vi "rsscope_core_global.vi"() -> ()   [LabVIEW 2014] (continued)
 "Access"=2, "Range Table"="rsscope_rngProtocolI2CRWBit", "Read Callback"="", "Write Callback"="", "Supported Models"="", "Instrument Options"="", "Flags"=0, "Help"="Defines if the R/W bit of a 7-bit address is considered separately or as part of the address.\n\nAvailable Repeated Capabilities:\nSerialBus: SB1, SB2, SB3, SB4\r\n\nRemote-control command(s):\nBUS<m>:I2C:RWBit"}, {"Level"=3, "Class Only"=FALSE, "Identifier"="RSSCOPE_ATTR_PROTOCOL_I2C_SELECTED_FRAME", "Descriptive Name"="Protocol I2C Selected Frame", "Data Type"=0, "Command"="", "Access"=2, "Range Table"="", "Read Callback"="", "Write Callback"="", "Supported Models"="", "Instrument Options"="", "Flags"=0, "Help"="Sets selector repeated capability Frame.\n\nAvailable Repeated Capabilities:\nNone\n\nRemote-control command(s):\ncmd"}, {"Level"=3, "Class Only"=FALSE, "Identifier"="RSSCOPE_ATTR_PROTOCOL_I2C_FRAME_COUNT", "Descriptive Name"="Protocol I2C Frame Count", "Data Type"=0, "Command"="BUS{SerialBus}:I2C:FCO?", "Access"=0, "Range Table"="", "Read Callback"="", "Write Callback"="", "Supported Models"="", "Instrument Options"="K0|K1", "Flags"=0, "Help"="Returns the number of decoded frames.\n\nAvailable Repeated Capabilities:\nSerialBus: SB1, SB2, SB3, SB4\r\n\nRemote-control command(s):\nBUS<m>:I2C:FCOunt?"}, {"Level"=3, "Class Only"=FALSE, "Identifier"="RSSCOPE_ATTR_PROTOCOL_I2C_FRAME_STATUS", "Descriptive Name"="Protocol I2C Frame Status", "Data Type"=0, "Command"="BUS{SerialBus}:I2C:FRAM<Frame>:STAT?", "Access"=0, "Range Table"="RsScope_rngI2CFrameStatus", "Read Callback"="rsscope_FormatI2CFrameRepCapInt32_ReadCallback.vi", "Write Callback"="", "Supported Models"="", "Instrument Options"="K1", "Flags"=0, "Help"="The overall state of the frame.\n\nAvailable Repeated Capabilities:\nSerialBus: SB1, SB2, SB3, SB4\r\n\nRemote-control command(s):\nBUS<m>:I2C:FRAMe<n>:STATus?"}, {"Level"=3, "Class Only"=FALSE, "Identifier"="RSSCOPE_ATTR_PROTOCOL_I2C_FRAME_START", "Descriptive Name"="Protocol I2C Frame Start", "Data Type"=1, "Command"="BUS{SerialBus}:I2C:FRAM<Frame>:STAR?", "Access"=0, "Range Table"="", "Read Callback"="rsscope_FormatI2CFrameRepCapReal64_ReadCallback.vi", "Write Callback"="", "Supported Models"="", "Instrument Options"="K1", "Flags"=0, "Help"="Return the start time of the selected frame.\n\nAvailable Repeated Capabilities:\nSerialBus: SB1, SB2, SB3, SB4\r\n\nRemote-control command(s):\nBUS<m>:I2C:FRAMe<n>:STARt?"}, {"Level"=3, "Class Only"=FALSE, "Identifier"="RSSCOPE_ATTR_PROTOCOL_I2C_FRAME_STOP", "Descriptive Name"="Protocol I2C Frame Stop", "Data Type"=1, "Command"="BUS{SerialBus}:I2C:FRAM<Frame>:STOP?", "Access"=0, "Range Table"="", "Read Callback"="rsscope_FormatI2CFrameRepCapReal64_ReadCallback.vi", "Write Callback"="", "Supported Models"="", "Instrument Options"="K1", "Flags"=0, "Help"="Return the stop time of the selected frame.\n\nAvailable Repeated Capabilities:\nSerialBus: SB1, SB2, SB3, SB4\r\n\nRemote-control command(s):\nBUS<m>:I2C:FRAMe<n>:STOP?"}, {"Level"=3, "Class Only"=FALSE, "Identifier"="RSSCOPE_ATTR_PROTOCOL_I2C_FRAME_ADDRESS_TYPE", "Descriptive Name"="Protocol I2C Frame Address Type", "Data Type"=0, "Command"="BUS{SerialBus}:I2C:FRAM<Frame>:AMOD?", "Access"=0, "Range Table"="RsScope_rngI2CFrameAddressType", "Read Callback"="rsscope_FormatI2CFrameRepCapInt32_ReadCallback.vi", "Write Callback"="", "Supported Models"="", "Instrument Options"="K1", "Flags"=0, "Help"="Returns the address length.\n\nAvailable Repeated Capabilities:\nSerialBus: SB1, SB2, SB3, SB4\r\n\nRemote-control command(s):\nBUS<m>:I2C:FRAMe<n>:AMODe?"}, {"Level"=3, "Class Only"=FALSE, "Identifier"="RSSCOPE_ATTR_PROTOCOL_I2C_FRAME_ADDRESS", "Descriptive Name"="Protocol I2C Frame Address", "Data Type"=0, "Command"="BUS{SerialBus}:I2C:FRAM<Frame>:ADDR?", "Access"=0, "Range Table"="", "Read Callback"="rsscope_FormatI2CFrameRepCapInt32_ReadCallback.vi", "Write Callback"="", "Supported Models"="", "Instrument Options"="K1", "Flags"=0, "Help"="Value of the frame address.\n\nAvailable Repeated Capabilities:\nSerialBus: SB1, SB2, SB3, SB4\r\n\nRemote-control command(s):\nBUS<m>:I2C:FRAMe<n>:ADDRess?"}, {"Level"=3, "Class Only"=FALSE, "Identifier"="RSSCOPE_ATTR_PROTOCOL_I2C_FRAME_RW_BIT", "Descriptive Name"="Protocol I2C Frame RW Bit", "Data Type"=0, "Command"="BUS{SerialBus}:I2C:FRAM<Frame>:ACC?", "Access"=0, "Range Table"="RsScope_rngI2CFrameRWBit", "Read Callback"="rsscope_FormatI2CFrameRepCapInt32_ReadCallback.vi", "Write Callback"="", "Supported Models"="", "Instrument Options"="K1", "Flags"=0, "Help"="Value of the R/W bit.\n\nAvailable Repeated Capabilities:\nSerialBus: SB1, SB2, SB3, SB4\r\n\nRemote-control command(s):\nBUS<m>:I2C:FRAMe<n>:ACCess?"}, {"Level"=3, "Class Only"=FALSE, "Identifier"="RSSCOPE_ATTR_PROTOCOL_I2C_FRAME_ACK_BIT", "Descriptive Name"="Protocol I2C Frame Ack Bit", "Data Type"=0, "Command"="BUS{SerialBus}:I2C:FRAM<Frame>:AACC?", "Access"=0, "Range Table"="RsScope_rngI2CFrameAckBit", "Read Callback"="rsscope_FormatI2CFrameRepCapInt32_ReadCallback.vi", "Write Callback"="", "Supported Models"="", "Instrument Options"="K1", "Flags"=0, "Help"="Value of the address acknowledge bit.\n\nAvailable Repeated Capabilities:\nSerialBus: SB1, SB2, SB3, SB4\r\n\nRemote-control command(s):\nBUS<m>:I2C:FRAMe<n>:AACCess?"}, {"Level"=3, "Class Only"=FALSE, "Identifier"="RSSCOPE_ATTR_PROTOCOL_I2C_FRAME_ACCESS_BIT_START", "Descriptive Name"="Protocol I2C Frame Access Bit Start", "Data Type"=1, "Command"="BUS{SerialBus}:I2C:FRAM<Frame>:RWBS?", "Access"=0, "Range Table"="", "Read Callback"="rsscope_FormatI2CFrameRepCapReal64_ReadCallback.vi", "Write Callback"="", "Supported Models"="", "Instrument Options"="K1", "Flags"=0, "Help"="Queries the start time of the access ack bit.\n\nAvailable Repeated Capabilities:\nSerialBus: SB1, SB2, SB3, SB4\r\n\nRemote-control command(s):\nBUS<m>:I2C:FRAMe<n>:RWBStart?"}, {"Level"=3, "Class Only"=FALSE, "Identifier"="RSSCOPE_ATTR_PROTOCOL_I2C_FRAME_SLAVE_ADDRESS", "Descriptive Name"="Protocol I2C Frame Slave Address", "Data Type"=0, "Command"="BUS{SerialBus}:I2C:FRAM<Frame>:ADEV?", "Access"=0, "Range Table"="", "Read Callback"="rsscope_FormatI2CFrameRepCapInt32_ReadCallback.vi", "Write Callback"="", "Supported Models"="", "Instrument Options"="K1", "Flags"=0, "Help"="Queries the slave address of the indicated frame.\n\nAvailable Repeated Capabilities:\nSerialBus: SB1, SB2, SB3, SB4\r\n\nRemote-control command(s):\nBUS<m>:I2C:FRAMe<n>:ADEVice?"}, {"Level"=3, "Class Only"=FALSE, "Identifier"="RSSCOPE_ATTR_PROTOCOL_I2C_FRAME_ADDRESS_START", "Descriptive Name"="Protocol I2C Frame Address Start", "Data Type"=1, "Command"="BUS{SerialBus}:I2C:FRAM<Frame>:AST?", "Access"=0, "Range Table"="", "Read Callback"="rsscope_FormatI2CFrameRepCapReal64_ReadCallback.vi", "Write Callback"="", "Supported Models"="", "Instrument Options"="K1", "Flags"=0, "Help"="Queries the start time of the address field for the indicated frame.\n\nAvailable Repeated Capabilities:\nSerialBus: SB1, SB2, SB3, SB4\r\n\nRemote-control command(s):\nBUS<m>:I2C:FRAMe<n>:ASTart?"}, {"Level"=3, "Class Only"=FALSE, "Identifier"="RSSCOPE_ATTR_PROTOCOL_I2C_FRAME_ADDRESS_ACK_BIT_START", "Descriptive Name"="Protocol I2C Frame Address Ack Bit Start", "Data Type"=1, "Command"="BUS{SerialBus}:I2C:FRAM<Frame>:ADBS?", "Access"=0, "Range Table"="", "Read Callback"="rsscope_FormatI2CFrameRepCapReal64_ReadCallback.vi", "Write Callback"="", "Supported Models"="", "Instrument Options"="K1", "Flags"=0, "Help"="Queries the start time of the address acknowledge bit.\n\nAvailable Repeated Capabilities:\nSerialBus: SB1, SB2, SB3, SB4\r\n\nRemote-control command(s):\nBUS<m>:I2C:FRAMe<n>:ADBStart?"}, {"Level"=3, "Class Only"=FALSE, "Identifier"="RSSCOPE_ATTR_PROTOCOL_I2C_FRAME_ADDRESS_COMPLETE", "Descriptive Name"="Protocol I2C Frame Address Complete", "Data Type"=3, "Command"="BUS{SerialBus}:I2C:FRAM<Frame>:ACOM?", "Access"=0, "Range Table"="", "Read Callback"="rsscope_FormatI2CFrameRepCapBoolean_ReadCallback.vi", "Write Callback"="", "Supported Models"="", "Instrument Options"="K1", "Flags"=0, "Help"="This function checks if address is complete.\n\nAvailable Repeated Capabilities:\nSerialBus: SB1, SB2, SB3, SB4\r\n\nRemote-control command(s):\nBUS<m>:I2C:FRAMe<n>:ACOMplete?"}, {"Level"=3, "Class Only"=FALSE, "Identifier"="RSSCOPE_ATTR_PROTOCOL_I2C_FRAME_BIT_RATE", "Descriptive Name"="Protocol I2C Frame Bit Rate", "Data Type"=5, "Command"="BUS{SerialBus}:I2C:FRAM<Frame>:BITR?", "Access"=0, "Range Table"="", "Read Callback"="rsscope_FormatI2CFrameRepCapInt64_ReadCallback.vi", "Write Callback"="", "Supported Models"="", "Instrument Options"="K1", "Flags"=0, "Help"="Returns the primary bit rate.\n\nAvailable Repeated Capabilities:\nSerialBus: SB1, SB2, SB3, SB4\r\n\nRemote-control command(s):\nBUS<m>:I2C:FRAMe<n>:BITRate?"}, {"Level"=3, "Class Only"=FALSE, "Identifier"="RSSCOPE_ATTR_PROTOCOL_I2C_FRAME_LENGTH", "Descriptive Name"="Protocol I2C Frame Length", "Data Type"=0, "Command"="BUS{SerialBus}:I2C:FRAM<Frame>:BCO?", "Access"=0, "Range Table"="", "Read Callback"="rsscope_FormatI2CFrameRepCapInt32_ReadCallback.vi", "Write Callback"="", "Supported Models"="", "Instrument Options"="K1", "Flags"=0, "Help"="This function returns the number of bytes in the specified frame.\n\nAvailable Repeated Capabilities:\nSerialBus: SB1, SB2, SB3, SB4\r\n\nRemote-control command(s):\nBUS<m>:I2C:FRAMe<n>:BCOunt?"}, {"Level"=3, "Class Only"=FALSE, "Identifier"="RSSCOPE_ATTR_PROTOCOL_I2C_FRAME_LABEL", "Descriptive Name"="Protocol I2C Frame Label", "Data Type"=2, "Command"="BUS{SerialBus}:I2C:FRAM<Frame>:SYMB?", "Access"=0, "Range Table"="", "Read Callback"="rsscope_FormatI2CFrameRepCapString_ReadCallback.vi", "Write Callback"="", "Supported Models"="", "Instrument Options"="K1", "Flags"=0, "Help"="This attribute returns the symbolic label of the specified frame if the label list is enabled.\n\nAvailable Repeated Capabilities:\nSerialBus: SB1, SB2, SB3, SB4\r\n\nRemote-control command(s):\nBUS<m>:I2C:FRAMe<n>:SYMBol?"}, {"Level"=3, "Class Only"=FALSE, "Identifier"="RSSCOPE_ATTR_PROTOCOL_I2C_SELECTED_BYTE", "Descriptive Name"="Protocol I2C Selected Byte", "Data Type"=0, "Command"="", "Access"=2, "Range Table"="", "Read Callback"="", "Write Callback"="", "Supported Models"="", "Instrument Options"="", "Flags"=0, "Help"="Sets selector repeated capability Byte.\n\nAvailable Repeated Capabilities:\nNone\n\nRemote-control command(s):\ncmd"}, {"Level"=3, "Class Only"=FALSE, "Identifier"="RSSCOPE_ATTR_PROTOCOL_I2C_FRAME_BYTE_DATA", "Descriptive Name"="Protocol I2C Frame Byte Data", "Data Type"=0, "Command"="BUS{SerialBus}:I2C:FRAM<Frame>:BYTE<Byte>:VAL?", "Access"=0, "Range Table"="", "Read Callback"="rsscope_FormatI2CByteRepCapInt32_ReadCallback.vi", "Write Callback"="", "Supported Models"="", "Instrument Options"="K1", "Flags"=0, "Help"="Value of the specified byte.\n\nAvailable Repeated Capabilities:\nSerialBus: SB1, SB2, SB3, SB4\r\n\nRemote-control command(s):\nBUS<m>:I2C:FRAMe<n>:BYTE<o>:VALue?"}, {"Level"=3, "Class Only"=FALSE, "Identifier"="RSSCOPE_ATTR_PROTOCOL_I2C_FRAME_BYTE_ACK_BIT_START", "Descriptive Name"="Protocol I2C Frame Byte Ack Bit Start", "Data Type"=1, "Command"="BUS{SerialBus}:I2C:FRAM<Frame>:BYTE<Byte>:ACKS?", "Access"=0, "Range Table"="", "Read Callback"="rsscope_FormatI2CByteRepCapReal64_ReadCallback.vi", "Write Callback"="", "Supported Models"="", "Instrument Options"="K1", "Flags"=0, "Help"="Returns the start time of the acknowledge bit of the specified byte.\n\nAvailable Repeated Capabilities:\nSerialBus: SB1, SB2, SB3, SB4\r\n\nRemote-control command(s):\nBUS<m>:I2C:FRAMe<n>:BYTE<o>:ACKStart?"}, {"Level"=3, "Class Only"=FALSE, "Identifier"="RSSCOPE_ATTR_PROTOCOL_I2C_FRAME_BYTE_START", "Descriptive Name"="Protocol I2C Frame Byte Start", "Data Type"=1, "Command"="BUS{SerialBus}:I2C:FRAM<Frame>:BYTE<Byte>:STAR?", "Access"=0, "Range Table"="", "Read Callback"="rsscope_FormatI2CByteRepCapReal64_ReadCallback.vi", "Write Callback"="", "Supported Models"="", "Instrument Options"="K1", "Flags"=0, "Help"="Queries the start time of the specified data byte.\n\nAvailable Repeated Capabilities:\nSerialBus: SB1, SB2, SB3, SB4\r\n\nRemote-control command(s):\nBUS<m>:I2C:FRAMe<n>:BYTE<o>:STARt?"}, {"Level"=3, "Class Only"=FALSE, "Identifier"="RSSCOPE_ATTR_PROTOCOL_I2C_FRAME_BYTE_ACK_BIT", "Descriptive Name"="Protocol I2C Frame Byte Ack Bit", "Data Type"=0, "Command"="BUS{SerialBus}:I2C:FRAM<Frame>:BYTE<Byte>:ACC?", "Access"=0, "Range Table"="RsScope_rngI2CFrameAckBit", "Read Callback"="rsscope_FormatI2CByteRepCapInt32_ReadCallback.vi", "Write Callback"="", "Supported Models"="", "Instrument Options"="K1", "Flags"=0, "Help"="Returns the acknowledge bit value of the specified data byte.\n\nAvailable Repeated Capabilities:\nSerialBus: SB1, SB2, SB3, SB4\r\n\nRemote-control command(s):\nBUS<m>:I2C:FRAMe<n>:BYTE<o>:ACCess?"}, {"Level"=3, "Class Only"=FALSE, "Identifier"="RSSCOPE_ATTR_PROTOCOL_I2C_FRAME_BYTE_COMPLETE", "Descriptive Name"="Protocol I2C Frame Byte Complete", "Data Type"=3, "Command"="BUS{SerialBus}:I2C:FRAM<Frame>:BYTE<Byte>:COMP?", "Access"=0, "Range Table"="", "Read Callback"="rsscope_FormatI2CByteRepCapBoolean_ReadCallback.vi", "Write Callback"="", "Supported Models"="", "Instrument Options"="K1", "Flags"=0, "Help"="Returns if the indicated byte is completely contained in the acquisition.\n\nAvailable Repeated Capabilities:\nSerialBus: SB1, SB2, SB3, SB4\r\n\nRemote-control command(s):\nBUS<m>:I2C:FRAMe<n>:BYTE<o>:COMPlete?"}, {"Level"=3, "Class Only"=TRUE, "Identifier"="", "Descriptive Name"="SCL", "Data Type"=0, "Command"="", "Access"=0, "Range Table"="", "Read Callback"="", "Write Callback"="", "Supported Models"="", "Instrument Options"="", "Flags"=0, "Help"="Configures I2C SCL properties."}, {"Level"=4, "Class Only"=FALSE, "Identifier"="RSSCOPE_ATTR_PROTOCOL_I2C_SCL_SOURCE", "Descriptive Name"="Protocol I2C SCL Source", "Data Type"=0, "Command"="BUS{SerialBus}:I2C:SCL:SOUR", "Access"=2, "Range Table"="rsscope_rngProtocolWaveformSource", "Read Callback"="", "Write Callback"="", "Supported Models"="", "Instrument Options"="", "Flags"=0, "Help"="Sets the waveform of the clock line.\n\nAvailable Repeated Capabilities:\nSerialBus: SB1, SB2, SB3, SB4\r\n\nRemote-control command(s):\nBUS<m>:I2C:SCL:SOURce"}, {"Level"=4, "Class Only"=FALSE, "Identifier"="RSSCOPE_ATTR_PROTOCOL_I2C_SCL_THRESHOLD", "Descriptive Name"="Protocol I2C SCL Threshold", "Data Type"=1, "Command"="BUS{SerialBus}:I2C:SCL:THR", "Access"=2, "Range Table"="rsscope_rngProtocolThreshold", "Read Callback"="", "Write Callback"="", "Supported Models"="", "Instrument Options"="", "Flags"=0, "Help"="Sets a user-defined threshold value for the clock line.\n\nAvailable Repeated Capabilities:\nSerialBus: SB1, SB2, SB3, SB4\r\n\nRemote-control command(s):\nBUS<m>:I2C:SCL:THReshold"}, {"Level"=3, "Class Only"=TRUE, "Identifier"="", "Descriptive Name"="SDA", "Data Type"=0, "Command"="", "Access"=0, "Range Table"="", "Read Callback"="", "Write Callback"="", "Supported Models"="", "Instrument Options"="", "Flags"=0, "Help"="Configures I2C SDA properties."}, {"Level"=4, "Class Only"=FALSE, "Identifier"="RSSCOPE_ATTR_PROTOCOL_I2C_SDA_SOURCE", "Descriptive Name"="Protocol I2C SDA Source", "Data Type"=0, "Command"="BUS{SerialBus}:I2C:SDA:SOUR", "Access"=2, "Range Table"="rsscope_rngProtocolWaveformSource", "Read Callback"="", "Write Callback"="", "Supported Models"="", "Instrument Options"="", "Flags"=0, "Help"="Sets the waveform of the data line.\n\nAvailable Repeated Capabilities:\nSerialBus: SB1, SB2, SB3, SB4\r\n\nRemote-control command(s):\nBUS<m>:I2C:SDA:SOURce"}, {"Level"=4, "Class Only"=FALSE, "Identifier"="RSSCOPE_ATTR_PROTOCOL_I2C_SDA_THRESHOLD", "Descriptive Name"="Protocol I2C SDA Threshold", "Data Type"=1, "Command"="BUS{SerialBus}:I2C:SDA:THR", "Access"=2, "Range Table"="rsscope_rngProtocolThreshold", "Read Callback"="", "Write Callback"="", "Supported Models"="", "Instrument Options"="", "Flags"=0, "Help"="Sets a user-defined threshold value for the data line.\n\nAvailable Repeated Capabilities:\nSerialBus: SB1, SB2, SB3, SB4\r\n\nRemote-control command(s):\nBUS<m>:I2C:SDA:THReshold"}, {"Level"=2, "Class Only"=TRUE, "Identifier"="", "Descriptive Name"="SPI", "Data Type"=0, "Command"="", "Access"=0, "Range Table"="", "Read Callback"="", "Write Callback"="", "Supported Models"="", "Instrument Options"="", "Flags"=0, "Help"="SPI (Serial Peripheral Interface) - decoding requires option R&S RTO-K1"}, {"Level"=3, "Class Only"=FALSE, "Identifier"="RSSCOPE_ATTR_PROTOCOL_SPI_BIT_ORDER", "Descriptive Name"="Protocol SPI Bit Order", "Data Type"=0, "Command"="BUS{SerialBus}:SPI:BORD", "Access"=2, "Range Table"="rsscope_rngProtocolSPIBitOrder", "Read Callback"="", "Write Callback"="", "Supported Models"="", "Instrument Options"="", "Flags"=0, "Help"="Defines if the data of the messages starts with msb (most significant bit) or lsb (least\n  significant bit).\n\nAvailable Repeated Capabilities:\nSerialBus: SB1, SB2, SB3, SB4\r\n\nRemote-control command(s):\nBUS<m>:SPI:BORDer"}, {"Level"=3, "Class Only"=FALSE, "Identifier"="RSSCOPE_ATTR_PROTOCOL_SPI_WORD_LENGTH", "Descriptive Name"="Protocol SPI Word Length", "Data Type"=0, "Command"="BUS{SerialBus}:SPI:WSIZ", "Access"=2, "Range Table"="rsscope_rngProtocolSPIWordLength", "Read Callback"="", "Write Callback"="", "Supported Models"="", "Instrument Options"="", "Flags"=0, "Help"="Sets the number of bits in a message.\n\nAvailable Repeated Capabilities:\nSerialBus: SB1, SB2, SB3, SB4\r\n\nRemote-control command(s):\nBUS<m>:SPI:WSIZe"}, {"Level"=3, "Class Only"=FALSE, "Identifier"="RSSCOPE_ATTR_PROTOCOL_SPI_TECHNOLOGY", "Descriptive Name"="Protocol SPI Technology", "Data Type"=0, "Command"="BUS{SerialBus}:SPI:TECH", "Access"=2, "Range Table"="rsscope_rngProtocolTechnology", "Read Callback"="", "Write Callback"="", "Supported Models"="", "Instrument Options"="", "Flags"=0, "Help"="Sets the threshold voltage clock and data lines as defined for various signal technologies.\n\nFor user defined values set to manual and use RSSCOPE_ATTR_PROTOCOL_SPI_THRESHOLD.\n\nAvailable Repeated Capabilities:\nSerialBus: SB1, SB2, SB3, SB4\r\n\nRemote-control command(s):\nBUS<m>:SPI:TECHnology"}, {"Level"=3, "Class Only"=FALSE, "Identifier"="RSSCOPE_ATTR_PROTOCOL_SPI_FRAME_START_CONDITION", "Descriptive Name"="Protocol SPI Frame Start Condition", "Data Type"=0, "Command"="BUS{SerialBus}:SPI:FRC", "Access"=2, "Range Table"="rsscope_rngProtocolSPIFrameStartCond", "Read Callback"="", "Write Callback"="", "Supported Models"="", "Instrument Options"="", "Flags"=0, "Help"="Select if frame start on Slave Select signal or on Clock line timeout defined by RSSCOPE_ATTR_PROTOCOL_SPI_FRAME_START_TIMEOUT\n\nAvailable Repeated Capabilities:\nSerialBus: SB1, SB2, SB3, SB4\r\n\nRemote-control command(s):\nBUS<m>:SPI:FRCondition"}, {"Level"=3, "Class Only"=FALSE, "Identifier"="RSSCOPE_ATTR_PROTOCOL_SPI_FRAME_START_TIMEOUT", "Descriptive Name"="Protocol SPI Frame Start Timeout", "Data Type"=1, "Command"="BUS{SerialBus}:SPI:TIM", "Access"=2, "Range Table"="rsscope_rngProtocolSPIFrameStartTimeout", "Read Callback"="", "Write Callback"="", "Supported Models"="", "Instrument Options"="", "Flags"=0, "Help"="Sets a timeout on the clock line SCLK as limiter between two frames.\n\nAvailable Repeated Capabilities:\nSerialBus: SB1, SB2, SB3, SB4\r\n\nRemote-control command(s):\nBUS<m>:SPI:TIMeout"}, {"Level"=3, "Class Only"=FALSE, "Identifier"="RSSCOPE_ATTR_PROTOCOL_SPI_SELECTED_FRAME", "Descriptive Name"="Protocol SPI Selected Frame", "Data Type"=0, "Command"="", "Access"=2, "Range Table"="", "Read Callback"="", "Write Callback"="", "Supported Models"="", "Instrument Options"="", "Flags"=0, "Help"="Sets selector repeated capability Frame.\n\nAvailable Repeated Capabilities:\nNone\n\nRemote-control command(s):\ncmd"}, {"Level"=3, "Class Only"=FALSE, "Identifier"="RSSCOPE_ATTR_PROTOCOL_SPI_FRAME_COUNT", "Descriptive Name"="Protocol SPI Frame Count", "Data Type"=0, "Command"="BUS{SerialBus}:SPI:FCOunt?", "Access"=0, "Range Table"="", "Read Callback"="", "Write Callback"="", "Supported Models"="", "Instrument Options"="K0|K1", "Flags"=0, "Help"="Returns the number of decoded frames.\n\nAvailable Repeated Capabilities:\nSerialBus: SB1, SB2, SB3, SB4\r\n\nRemote-control command(s):\nBUS<m>:SPI:FCOunt?"}, {"Level"=3, "Class Only"=FALSE, "Identifier"="RSSCOPE_ATTR_PROTOCOL_SPI_FRAME_WORD_COUNT", "Descriptive Name"="Protocol SPI Frame Word Count", "Data Type"=0, "Command"="BUS{SerialBus}:SPI:FRAM<Frame>:WCO?", "Access"=0, "Range Table"="", "Read Callback"="rsscope_FormatSPIFrameRepCapInt32_ReadCallback.vi", "Write Callback"="", "Supported Models"="", "Instrument Options"="K1", "Flags"=0, "Help"="Queries the number of words in frame.\n\nAvailable Repeated Capabilities:\nSerialBus: SB1, SB2, SB3, SB4\r\n\nRemote-control command(s):\nBUS<m>:SPI:FRAMe<n>:WCOunt?"}, {"Level"=3, "Class Only"=FALSE, "Identifier"="RSSCOPE_ATTR_PROTOCOL_SPI_FRAME_START", "Descriptive Name"="Protocol SPI Frame Start", "Data Type"=1, "Command"="BUS{SerialBus}:SPI:FRAM<Frame>:STAR?", "Access"=0, "Range Table"="", "Read Callback"="rsscope_FormatSPIFrameRepCapReal64_ReadCallback.vi", "Write Callback"="", "Supported Models"="", "Instrument Options"="K1", "Flags"=0, "Help"="Return the start time of the selected frame.\n\nAvailable Repeated Capabilities:\nSerialBus: SB1, SB2, SB3, SB4\r\n\nRemote-control command(s):\nBUS<m>:SPI:FRAMe<n>:STARt?"}, {"Level"=3, "Class Only"=FALSE, "Identifier"="RSSCOPE_ATTR_PROTOCOL_SPI_FRAME_STOP", "Descriptive Name"="Protocol SPI Frame Stop", "Data Type"=1, "Command"="BUS{SerialBus}:SPI:FRAM<Frame>:STOP?", "Access"=0, "Range Table"="", "Read Callback"="rsscope_FormatSPIFrameRepCapReal64_ReadCallback.vi", "Write Callback"="", "Supported Models"="", "Instrument Options"="K1", "Flags"=0, "Help"="Return the stop time of the selected frame.\n\nAvailable Repeated Capabilities:\nSerialBus: SB1, SB2, SB3, SB4\r\n\nRemote-control command(s):\nBUS<m>:SPI:FRAMe<n>:STOP?"}, {"Level"=3, "Class Only"=FALSE, "Identifier"="RSSCOPE_ATTR_PROTOCOL_SPI_FRAME_BIT_RATE", "Descriptive Name"="Protocol SPI Frame Bit Rate", "Data Type"=5, "Command"="BUS{SerialBus}:SPI:FRAM<Frame>:BITR?", "Access"=0, "Range Table"="", "Read Callback"="rsscope_FormatSPIFrameRepCapInt64_ReadCallback.vi", "Write Callback"="", "Supported Models"="", "Instrument Options"="", "Flags"=0, "Help"="Returns the primary bit rate.\n\nAvailable Repeated Capabilities:\nSerialBus: SB1, SB2, SB3, SB4\r\n\nRemote-control command(s):\nBUS<m>:SPI:FRAMe<n>:BITRate?"}, {"Level"=3, "Class Only"=FALSE, "Identifier"="RSSCOPE_ATTR_PROTOCOL_SPI_FRAME_STATUS", "Descriptive Name"="Protocol SPI Frame Status", "Data Type"=0, "Command"="BUS{SerialBus}:SPI:FRAM<Frame>:STAT?", "Access"=0, "Range Table"="RsScope_rngSPIFrameStatus", "Read Callback"="rsscope_FormatSPIFrameRepCapInt32_ReadCallback.vi", "Write Callback"="", "Supported Models"="", "Instrument Options"="K1", "Flags"=0, "Help"="The overall state of the frame.\n\nAvailable Repeated Capabilities:\nSerialBus: SB1, SB2, SB3, SB4\r\n\nRemote-control command(s):\nBUS<m>:SPI:FRAMe<n>:STATus?"}, {"Level"=3, "Class Only"=FALSE, "Identifier"="RSSCOPE_ATTR_PROTOCOL_SPI_SELECTED_WORD", "Descriptive Name"="Protocol SPI Selected Word", "Data Type"=0, "Command"="", "Access"=2, "Range Table"="", "Read Callback"="", "Write Callback"="", "Supported Models"="", "Instrument Options"="", "Flags"=0, "Help"="Sets selector repeated capability Word.\n\nAvailable Repeated Capabilities:\nNone\n\nRemote-control command(s):\ncmd"}, {"Level"=3, "Class Only"=FALSE, "Identifier"="RSSCOPE_ATTR_PROTOCOL_SPI_FRAME_WORD_START", "Descriptive Name"="Protocol SPI Frame Word Start", "Data Type"=1, "Command"="BUS{SerialBus}:SPI:FRAM<Frame>:WORD<Word>:STAR?", "Access"=0, "Range Table"="", "Read Callback"="rsscope_FormatSPIWordRepCapReal64_ReadCallback.vi", "Write Callback"="", "Supported Models"="", "Instrument Options"="K1", "Flags"=0, "Help"="Start time of the data word.\n\nAvailable Repeated Capabilities:\nSerialBus: SB1, SB2, SB3, SB4\r\n\nRemote-control command(s):\nBUS<m>:SPI:FRAMe<n>:WORD<o>:STARt?"}, {"Level"=3, "Class Only"=FALSE, "Identifier"="RSSCOPE_ATTR_PROTOCOL_SPI_FRAME_WORD_STOP", "Descriptive Name"="Protocol SPI Frame Word Stop", "Data Type"=1, "Command"="BUS{SerialBus}:SPI:FRAM<Frame>:WORD<Word>:STOP?", "Access"=0, "Range Table"="", "Read Callback"="rsscope_FormatSPIWordRepCapReal64_ReadCallback.vi", "Write Callback"="", "Supported Models"="", "Instrument Options"="K1", "Flags"=0, "Help"="Stop time of the data word.\n\nAvailable Repeated Capabilities:\nSerialBus: SB1, SB2, SB3, SB4\r\n\nRemote-control command(s):\nBUS<m>:SPI:FRAMe<n>:WORD<o>:STOP?"}, {"Level"=3, "Class Only"=FALSE, "Identifier"="RSSCOPE_ATTR_PROTOCOL_SPI_FRAME_WORD_MISO", "Descriptive Name"="Protocol SPI Frame Word MISO", "Data Type"=0, "Command"="BUS{SerialBus}:SPI:FRAM<Frame>:WORD<Word>:MISO?", "Access"=0, "Range Table"="", "Read Callback"="rsscope_FormatSPIWordRepCapInt32_ReadCallback.vi", "Write Callback"="", "Supported Models"="", "Instrument Options"="K1", "Flags"=0, "Help"="Returns the data value of the specified word on the MISO line.\n\nAvailable Repeated Capabilities:\nSerialBus: SB1, SB2, SB3, SB4\r\n\nRemote-control command(s):\nBUS<m>:SPI:FRAMe<n>:WORD<o>:MISO?"}, {"Level"=3, "Class Only"=FALSE, "Identifier"="RSSCOPE_ATTR_PROTOCOL_SPI_FRAME_WORD_MISO_FORMATTED_VALUE", "Descriptive Name"="Protocol SPI Frame Word MISO Formatted Value", "Data Type"=2, "Command"="BUS{SerialBus}:SPI:FRAM<Frame>:WORD<Word>:FMIS?", "Access"=0, "Range Table"="", "Read Callback"="rsscope_FormatSPIWordRepCapString_ReadCallback.vi", "Write Callback"="", "Supported Models"="", "Instrument Options"="K1", "Flags"=0, "Help"="Returns the formatted value of the specified word on the MISO line.\n\nAvailable Repeated Capabilities:\nSerialBus: SB1, SB2, SB3, SB4\r\n\nRemote-control command(s):\nBUS<m>:SPI:FRAMe<n>:WORD<o>:FMISo?"}, {"Level"=3, "Class Only"=FALSE, "Identifier"="RSSCOPE_ATTR_PROTOCOL_SPI_FRAME_WORD_MOSI", "Descriptive Name"="Protocol SPI Frame Word MOSI", "Data Type"=0, "Command"="BUS{SerialBus}:SPI:FRAM<Frame>:WORD<Word>:MOSI?", "Access"=0, "Range Table"="", "Read Callback"="rsscope_FormatSPIWordRepCapInt32_ReadCallback.vi", "Write Callback"="", "Supported Models"="", "Instrument Options"="K1", "Flags"=0, "Help"="Returns the data value of the specified word on the MOSI line.\n\nAvailable Repeated Capabilities:\nSerialBus: SB1, SB2, SB3, SB4\r\n\nRemote-control command(s):\nBUS<m>:SPI:FRAMe<n>:WORD<o>:MOSI?"}, {"Level"=3, "Class Only"=FALSE, "Identifier"="RSSCOPE_ATTR_PROTOCOL_SPI_FRAME_WORD_MOSI_FORMATTED_VALUE", "Descriptive Name"="Protocol SPI Frame Word MOSI Formatted Value", "Data Type"=2, "Command"="BUS{SerialBus}:SPI:FRAM<Frame>:WORD<Word>:FMOS?", "Access"=0, "Range Table"="", "Read Callback"="rsscope_FormatSPIWordRepCapString_ReadCallback.vi", "Write Callback"="", "Supported Models"="", "Instrument Options"="K1", "Flags"=0, "Help"="Returns the formatted value of the specified word on the MOSI line.\n\nAvailable Repeated Capabilities:\nSerialBus: SB1, SB2, SB3, SB4\r\n\nRemote-control command(s):\nBUS<m>:SPI:FRAMe<n>:WORD<o>:FMOSi?"}, {"Level"=3, "Class Only"=TRUE, "Identifier"="", "Descriptive Name"="Clock", "Data Type"=0, "Command"="", "Access"=0, "Range Table"="", "Read Callback"="", "Write Callback"="", "Supported Models"="", "Instrument Options"="", "Flags"=0, "Help"="Configures SPI Clock properties."}, {"Level"=4, "Class Only"=FALSE, "Identifier"="RSSCOPE_ATTR_PROTOCOL_SPI_CLOCK_SOURCE", "Descriptive Name"="Protocol SPI Clock Source", "Data Type"=0, "Command"="BUS{SerialBus}:SPI:SCLK:SOUR", "Access"=2, "Range Table"="rsscope_rngProtocolWaveformSource", "Read Callback"="", "Write Callback"="", "Supported Models"="", "Instrument Options"="", "Flags"=0, "Help"="Sets the input channel of the clock line.\n\nAvailable Repeated Capabilities:\nSerialBus: SB1, SB2, SB3, SB4\r\n\nRemote-control command(s):\nBUS<m>:SPI:SCLK:SOURce"}, {"Level"=4, "Class Only"=FALSE, "Identifier"="RSSCOPE_ATTR_PROTOCOL_SPI_CLOCK_THRESHOLD", "Descriptive Name"="Protocol SPI Clock Threshold", "Data Type"=1, "Command"="BUS{SerialBus}:SPI:SCLK:THR", "Access"=2, "Range Table"="rsscope_rngProtocolThreshold", "Read Callback"="", "Write Callback"="", "Supported Models"="", "Instrument Options"="", "Flags"=0, "Help"="Set user-defined threshold values for the clock lines.\n\nAvailable Repeated Capabilities:\nSerialBus: SB1, SB2, SB3, SB4\r\n\nRemote-control command(s):\nBUS<m>:SPI:SCLK:THReshold"}, {"Level"=3, "Class Only"=TRUE, "Identifier"="", "Descriptive Name"="MOSI", "Data Type"=0, "Command"="", "Access"=0, "Range Table"="", "Read Callback"="", "Write Callback"="", "Supported Models"="", "Instrument Options"="", "Flags"=0, "Help"="Configures SPI MOSI properties."}, {"Level"=4, "Class Only"=FALSE, "Identifier"="RSSCOPE_ATTR_PROTOCOL_SPI_MOSI_SOURCE", "Descriptive Name"="Protocol SPI MOSI Source", "Data Type"=0, "Command"="BUS{SerialBus}:SPI:MOSI:SOUR", "Access"=2, "Range Table"="rsscope_rngProtocolWaveformSource", "Read Callback"="", "Write Callback"="", "Supported Models"="", "Instrument Options"="", "Flags"=0, "Help"="Sets the input channel of the MOSI line.\n\nAvailable Repeated Capabilities:\nSerialBus: SB1, SB2, SB3, SB4\r\n\nRemote-control command(s):\nBUS<m>:SPI:MOSI:SOURce"}, {"Level"=4, "Class Only"=FALSE, "Identifier"="RSSCOPE_ATTR_PROTOCOL_SPI_MOSI_POLARITY", "Descriptive Name"="Protocol SPI MOSI Polarity", "Data Type"=0, "Command"="BUS{SerialBus}:SPI:MOSI:POL", "Access"=2, "Range Table"="rsscope_rngProtocolSPIPolarity", "Read Callback"="", "Write Callback"="", "Supported Models"="", "Instrument Options"="", "Flags"=0, "Help"="Selects whether transmitted data is high active (high = 1) or low active (low = 1).\n\nAvailable Repeated Capabilities:\nSerialBus: SB1, SB2, SB3, SB4\r\n\nRemote-control command(s):\nBUS<m>:SPI:MOSI:POLarity"}, {"Level"=4, "Class Only"=FALSE, "Identifier"="RSSCOPE_ATTR_PROTOCOL_SPI_MOSI_THRESHOLD", "Descriptive Name"="Protocol SPI MOSI Threshold", "Data Type"=1, "Command"="BUS{SerialBus}:SPI:MOSI:THR", "Access"=2, "Range Table"="rsscope_rngProtocolThreshold", "Read Callback"="", "Write Callback"="", "Supported Models"="", "Instrument Options"="", "Flags"=0, "Help"="Set user-defined threshold values for the MOSI lines.\n\nAvailable Repeated Capabilities:\nSerialBus: SB1, SB2, SB3, SB4\r\n\nRemote-control command(s):\nBUS<m>:SPI:MOSI:THReshold"}, {"Level"=3, "Class Only"=TRUE, "Identifier"="", "Descriptive Name"="MISO", "Data Type"=0, "Command"="", "Access"=0, "Range Table"="", "Read Callback"="", "Write Callback"="", "Supported Models"="", "Instrument Options"="", "Flags"=0, "Help"="Configures SPI MISO properties."}, {"Level"=4, "Class Only"=FALSE, "Identifier"="RSSCOPE_ATTR_PROTOCOL_SPI_MISO_SOURCE", "Descriptive Name"="Protocol SPI MISO Source", "Data Type"=0, "Command"="BUS{SerialBus}:SPI:MISO:SOUR", "Access"=2, "Range Table"="rsscope_rngProtocolWaveformSource", "Read Callback"="", "Write Callback"="", "Supported Models"="", "Instrument Options"="", "Flags"=0, "Help"="Sets the input channel of the MISO line.\n\nAvailable Repeated Capabilities:\nSerialBus: SB1, SB2, SB3, SB4\r\n\nRemote-control command(s):\nBUS<m>:SPI:MISO:SOURce"}, {"Level"=4, "Class Only"=FALSE, "Identifier"="RSSCOPE_ATTR_PROTOCOL_SPI_MISO_POLARITY", "Descriptive Name"="Protocol SPI MISO Polarity", "Data Type"=0, "Command"="BUS{SerialBus}:SPI:MISO:POL", "Access"=2, "Range Table"="rsscope_rngProtocolSPIPolarity", "Read Callback"="", "Write Callback"="", "Supported Models"="", "Instrument Options"="", "Flags"=0, "Help"="Selects whether transmitted data is high active (high = 1) or low active (low = 1).\n\nAvailable Repeated Capabilities:\nSerialBus: SB1, SB2, SB3, SB4\r\n\nRemote-control command(s):\nBUS<m>:SPI:MISO:POLarity"}, {"Level"=4, "Class Only"=FALSE, "Identifier"="RSSCOPE_ATTR_PROTOCOL_SPI_MISO_THRESHOLD", "Descriptive Name"="Protocol SPI MISO Threshold", "Data Type"=1, "Command"="BUS{SerialBus}:SPI:MISO:THR", "Access"=2, "Range Table"="rsscope_rngProtocolThreshold", "Read Callback"="", "Write Callback"="", "Supported Models"="", "Instrument Options"="", "Flags"=0, "Help"="Set user-defined threshold values for the MISO lines.\n\nAvailable Repeated Capabilities:\nSerialBus: SB1, SB2, SB3, SB4\r\n\nRemote-control command(s):\nBUS<m>:SPI:MISO:THReshold"}, {"Level"=3, "Class Only"=TRUE, "Identifier"="", "Descriptive Name"="Slave Select", "Data Type"=0, "Command"="", "Access"=0, "Range Table"="", "Read Callback"="", "Write Callback"="", "Supported Models"="", "Instrument Options"="", "Flags"=0, "Help"="Configures SPI Slave Select properties."}, {"Level"=4, "Class Only"=FALSE, "Identifier"="RSSCOPE_ATTR_PROTOCOL_SPI_SLAVE_SELECT_SOURCE", "Descriptive Name"="Protocol SPI Slave Select Source", "Data Type"=0, "Command"="BUS{SerialBus}:SPI:SSEL:SOUR", "Access"=2, "Range Table"="rsscope_rngProtocolWaveformSource", "Read Callback"="", "Write Callback"="", "Supported Models"="", "Instrument Options"="", "Flags"=0, "Help"="Sets the input channel of the Slave Select line.\n\nAvailable Repeated Capabilities:\nSerialBus: SB1, SB2, SB3, SB4\r\n\nRemote-control command(s):\nBUS<m>:SPI:SSELect:SOURce"}, {"Level"=4, "Class Only"=FALSE, "Identifier"="RSSCOPE_ATTR_PROTOCOL_SPI_SLAVE_SELECT_POLARITY", "Descriptive Name"="Protocol SPI Slave Select Polarity", "Data Type"=0, "Command"="BUS{SerialBus}:SPI:SSEL:POL", "Access"=2, "Range Table"="rsscope_rngProtocolSPIPolarity", "Read Callback"="", "Write Callback"="", "Supported Models"="", "Instrument Options"="", "Flags"=0, "Help"="Selects whether transmitted slave select signal is high active (high = 1) or low active (low = 1).\n\nAvailable Repeated Capabilities:\nSerialBus: SB1, SB2, SB3, SB4\r\n\nRemote-control command(s):\nBUS<m>:SPI:SSELect:POLarity"}, {"Level"=4, "Class Only"=FALSE, "Identifier"="RSSCOPE_ATTR_PROTOCOL_SPI_SLAVE_SELECT_THRESHOLD", "Descriptive Name"="Protocol SPI Slave Select Threshold", "Data Type"=1, "Command"="BUS{SerialBus}:SPI:SSEL:THR", "Access"=2, "Range Table"="rsscope_rngProtocolThreshold", "Read Callback"="", "Write Callback"="", "Supported Models"="", "Instrument Options"="", "Flags"=0, "Help"="Set user-defined threshold values for the slave select lines.\n\nAvailable Repeated Capabilities:\nSerialBus: SB1, SB2, SB3, SB4\r\n\nRemote-control command(s):\nBUS<m>:SPI:SSELect:THReshold"}, {"Level"=2, "Class Only"=TRUE, "Identifier"="", "Descriptive Name"="UART", "Data Type"=0, "Command"="", "Access"=0, "Range Table"="", "Read Callback"="", "Write Callback"="", "Supported Models"="", "Instrument Options"="", "Flags"=0, "Help"="UART/RS232 (EIA-232 serial interface) - decoding requires option R&S RTO-K2"}, {"Level"=3, "Class Only"=FALSE, "Identifier"="RSSCOPE_ATTR_PROTOCOL_UART_TECHNOLOGY", "Descriptive Name"="Protocol UART Technology", "Data Type"=0, "Command"="BUS{SerialBus}:UART:TECH", "Access"=2, "Range Table"="rsscope_rngProtocolTechnology", "Read Callback"="", "Write Callback"="", "Supported Models"="", "Instrument Options"="", "Flags"=0, "Help"="Sets the threshold voltage Tx and Rx lines as defined for various signal technologies.\n\nFor user defined values set to manual and use RSSCOPE_ATTR_PROTOCOL_UART_THRESHOLD.\n\nAvailable Repeated Capabilities:\nSerialBus: SB1, SB2, SB3, SB4\r\n\nRemote-control command(s):\nBUS<m>:UART:TECHnology"}, {"Level"=3, "Class Only"=FALSE, "Identifier"="RSSCOPE_ATTR_PROTOCOL_UART_BIT_RATE", "Descriptive Name"="Protocol UART Bit Rate", "Data Type"=0, "Command"="BUS{SerialBus}:UART:BAUD", "Access"=2, "Range Table"="rsscope_rngProtocolUARTBitRate", "Read Callback"="", "Write Callback"="", "Supported Models"="", "Instrument Options"="", "Flags"=0, "Help"="Sets the number of transmitted bits per second.\n\nAvailable Repeated Capabilities:\nSerialBus: SB1, SB2, SB3, SB4\r\n\nRemote-control command(s):\nBUS<m>:UART:BAUDrate"}, {"Level"=3, "Class Only"=FALSE, "Identifier"="RSSCOPE_ATTR_PROTOCOL_UART_PARITY", "Descriptive Name"="Protocol UART Parity", "Data Type"=0, "Command"="BUS{SerialBus}:UART:PAR", "Access"=2, "Range Table"="rsscope_rngProtocolUARTParity", "Read Callback"="", "Write Callback"="", "Supported Models"="", "Instrument Options"="", "Flags"=0, "Help"="Defines the optional parity bit that is used for error detection.\n\nAvailable Repeated Capabilities:\nSerialBus: SB1, SB2, SB3, SB4\r\n\nRemote-control command(s):\nBUS<m>:UART:PARity"}, {"Level"=3, "Class Only"=FALSE, "Identifier"="RSSCOPE_ATTR_PROTOCOL_UART_POLARITY", "Descriptive Name"="Protocol UART Polarity", "Data Type"=0, "Command"="BUS{SerialBus}:UART:POL", "Access"=2, "Range Table"="rsscope_rngProtocolPolarity", "Read Callback"="", "Write Callback"="", "Supported Models"="", "Instrument Options"="", "Flags"=0, "Help"="Defines if the transmitted data on the bus is high (high = 1) or low (low = 1) active.\n\nAvailable Repeated Capabilities:\nSerialBus: SB1, SB2, SB3, SB4\r\n\nRemote-control command(s):\nBUS<m>:UART:POLarity"}, {"Level"=3, "Class Only"=FALSE, "Identifier"="RSSCOPE_ATTR_PROTOCOL_UART_STOP_BITS", "Descriptive Name"="Protocol UART Stop Bits", "Data Type"=0, "Command"="BUS{SerialBus}:UART:SBIT", "Access"=2, "Range Table"="rsscope_rngProtocolUARTStopBits", "Read Callback"="", "Write Callback"="", "Supported Models"="", "Instrument Options"="", "Flags"=0, "Help"="Sets the number of stop bits: 1; 1.5 or 2 stop bits are possible.\n\nAvailable Repeated Capabilities:\nSerialBus: SB1, SB2, SB3, SB4\r\n\nRemote-control command(s):\nBUS<m>:UART:SBIT"}, {"Level"=3, "Class Only"=FALSE, "Identifier"="RSSCOPE_ATTR_PROTOCOL_UART_DATA_BITS_COUNT", "Descriptive Name"="Protocol UART Data Bits Count", "Data Type"=0, "Command"="BUS{SerialBus}:UART:SSIZ", "Access"=2, "Range Table"="rsscope_rngProtocolUARTDataBitsCount", "Read Callback"="", "Write Callback"="", "Supported Models"="", "Instrument Options"="", "Flags"=0, "Help"="Sets the number of data bits in a message.\n\nAvailable Repeated Capabilities:\nSerialBus: SB1, SB2, SB3, SB4\r\n\nRemote-control command(s):\nBUS<m>:UART:SSIZe"}, {"Level"=3, "Class Only"=FALSE, "Identifier"="RSSCOPE_ATTR_PROTOCOL_UART_WORD_COUNT", "Descriptive Name"="Protocol UART Word Count", "Data Type"=0, "Command"="BUS{SerialBus}:UART:WORD:COUN?", "Access"=0, "Range Table"="", "Read Callback"="", "Write Callback"="", "Supported Models"="", "Instrument Options"="K0|K2", "Flags"=0, "Help"="Returns the number of words in the acquisition.\n\nAvailable Repeated Capabilities:\nSerialBus: SB1, SB2, SB3, SB4\r\n\nRemote-control command(s):\nBUS<m>:UART:WORD<n>:COUNt?"}, {"Level"=3, "Class Only"=FALSE, "Identifier"="RSSCOPE_ATTR_PROTOCOL_UART_PRIMARY_BIT_RATE", "Descriptive Name"="Protocol UART Primary Bit Rate", "Data Type"=5, "Command"="BUS{SerialBus}:UART:WORD1:BITR?", "Access"=0, "Range Table"="", "Read Callback"="", "Write Callback"="", "Supported Models"="", "Instrument Options"="", "Flags"=0, "Help"="Returns the primary bit rate.\n\nAvailable Repeated Capabilities:\nSerialBus: SB1, SB2, SB3, SB4\r\n\nRemote-control command(s):\nBUS<m>:UART:WORD<n>:BITRate?"}, {"Level"=3, "Class Only"=FALSE, "Identifier"="RSSCOPE_ATTR_PROTOCOL_UART_PACKETS", "Descriptive Name"="Protocol UART Packets", "Data Type"=0, "Command"="BUS{SerialBus}:UART:PACK", "Access"=2, "Range Table"="rsscope_rngProtocolPackets", "Read Callback"="", "Write Callback"="", "Supported Models"="", "Instrument Options"="", "Flags"=0, "Help"="Defines the method of packet separation. A packet is a number of subsequent words in a date stream.\n\nAvailable Repeated Capabilities:\nSerialBus: SB1, SB2, SB3, SB4\r\n\nRemote-control command(s):\nBUS<m>:UART:PACKets"}, {"Level"=3, "Class Only"=FALSE, "Identifier"="RSSCOPE_ATTR_PROTOCOL_UART_TOUT", "Descriptive Name"="Protocol UART Tout", "Data Type"=1, "Command"="BUS{SerialBus}:UART:TOUT", "Access"=2, "Range Table"="rsscope_rngProtocolUARTInterframeTime", "Read Callback"="", "Write Callback"="", "Supported 
